vi "Data to Plot.vi"(6 "Array 3":dbl[][](array[numeric]), 9 "Array of Double":dbl[](array[numeric]), 10 "Array of Double 2":dbl[](array[numeric]), 11 "Arrow":dbl[](array[numeric])) -> (1 "Cluster 2":cluster{dbl[], dbl[]}, 2 "Cluster 3":cluster{dbl[], dbl[]}, 3 "Cluster 4":cluster{dbl[], dbl[]}, 4 "Cluster":cluster{dbl[], dbl[]}, 5 "Array 2":dbl[](array[numeric]), 7 "Array":dbl[](array[numeric]))   [LabVIEW 2021]
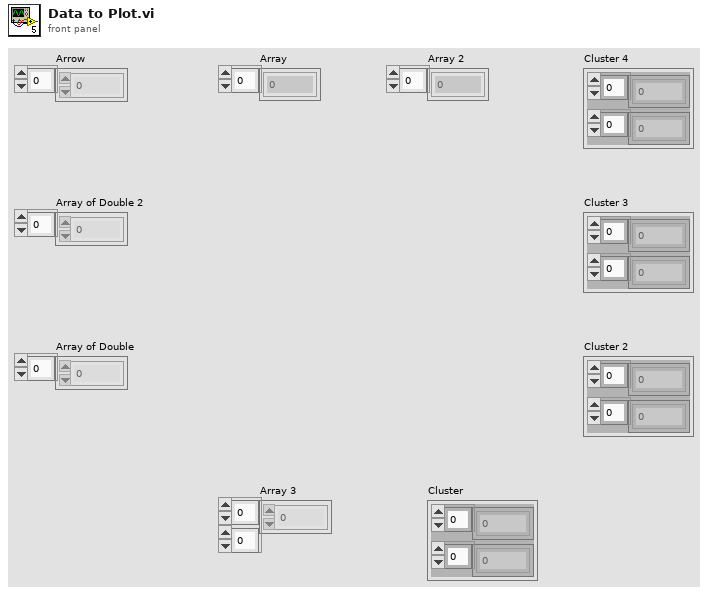
[diagram p1: front panel]
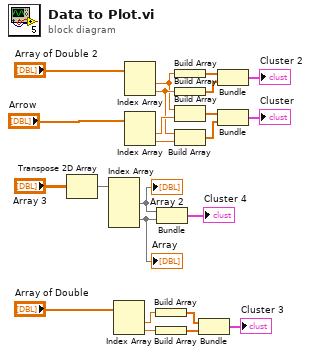
[diagram p0: block diagram]
diagram:
  n1 = Transpose 2D Array(2D array="Array 3") -> (transposed array=w13:dbl[][])
  n2 = Index Array(array=w13) -> (element #1=w9:dbl[], element #2=w10:dbl[])  [unwired: 4 in]
  "Array" <- w10
  "Array 2" <- w9
  n3 = Index Array(array="Array of Double") -> (element #1=w15:dbl, element #2=w14:dbl)  [unwired: 2 in]
  n4 = Index Array(array="Array of Double 2") -> (element #1=w18:dbl, element #2=w19:dbl)  [unwired: 2 in]
  n5 = Index Array(array="Arrow") -> (element #1=w22:dbl, element #2=w23:dbl)  [unwired: 2 in]
  n6 = Build Array(w15) -> (w11:dbl[])
  n7 = Build Array(w14) -> (w12:dbl[])
  n8 = Bundle(w9, w10) -> (→"Cluster 4":cluster{dbl[], dbl[]})  [unwired: 1 in]
  n9 = Build Array(w18) -> (w16:dbl[])
  n10 = Build Array(w19) -> (w17:dbl[])
  n11 = Build Array(w18, w22) -> (w20:dbl[])
  n12 = Build Array(w19, w23) -> (w21:dbl[])
  n13 = Bundle(w11, w12) -> (→"Cluster 3":cluster{dbl[], dbl[]})  [unwired: 1 in]
  n14 = Bundle(w16, w17) -> (→"Cluster 2":cluster{dbl[], dbl[]})  [unwired: 1 in]
  n15 = Bundle(w20, w21) -> (→"Cluster":cluster{dbl[], dbl[]})  [unwired: 1 in]
